vi "Diff Configuration.vi"(8 "error in":errorcluster, 10 "configuration new":T4[](array[typedef]), 11 "configuration old":T4[](array[typedef])) -> (0 "error out":errorcluster, 3 "configuration diff":T1[](array[typedef]))   [LabVIEW 2020, in "Ballard MIL-STD-1553 System Explorer.lvlib" / "Implementation.lvlib" / "Refresh.lvlib"]
uses:
  Refresh.lvlib
  Change Type.ctl
  Symbols.ctl
  MCL Row.ctl
  Scripting/Constants.vi
  Scripting/Ballard MIL-STD-1553 Scripting.lvlib
  Shared/Address.ctl
  Shared/Message Type.ctl
  Shared/Terminal Endpoint.ctl
  Shared/Parameter Definition.ctl
  Shared/Message Definition.ctl
  Shared/1553 Channel.ctl
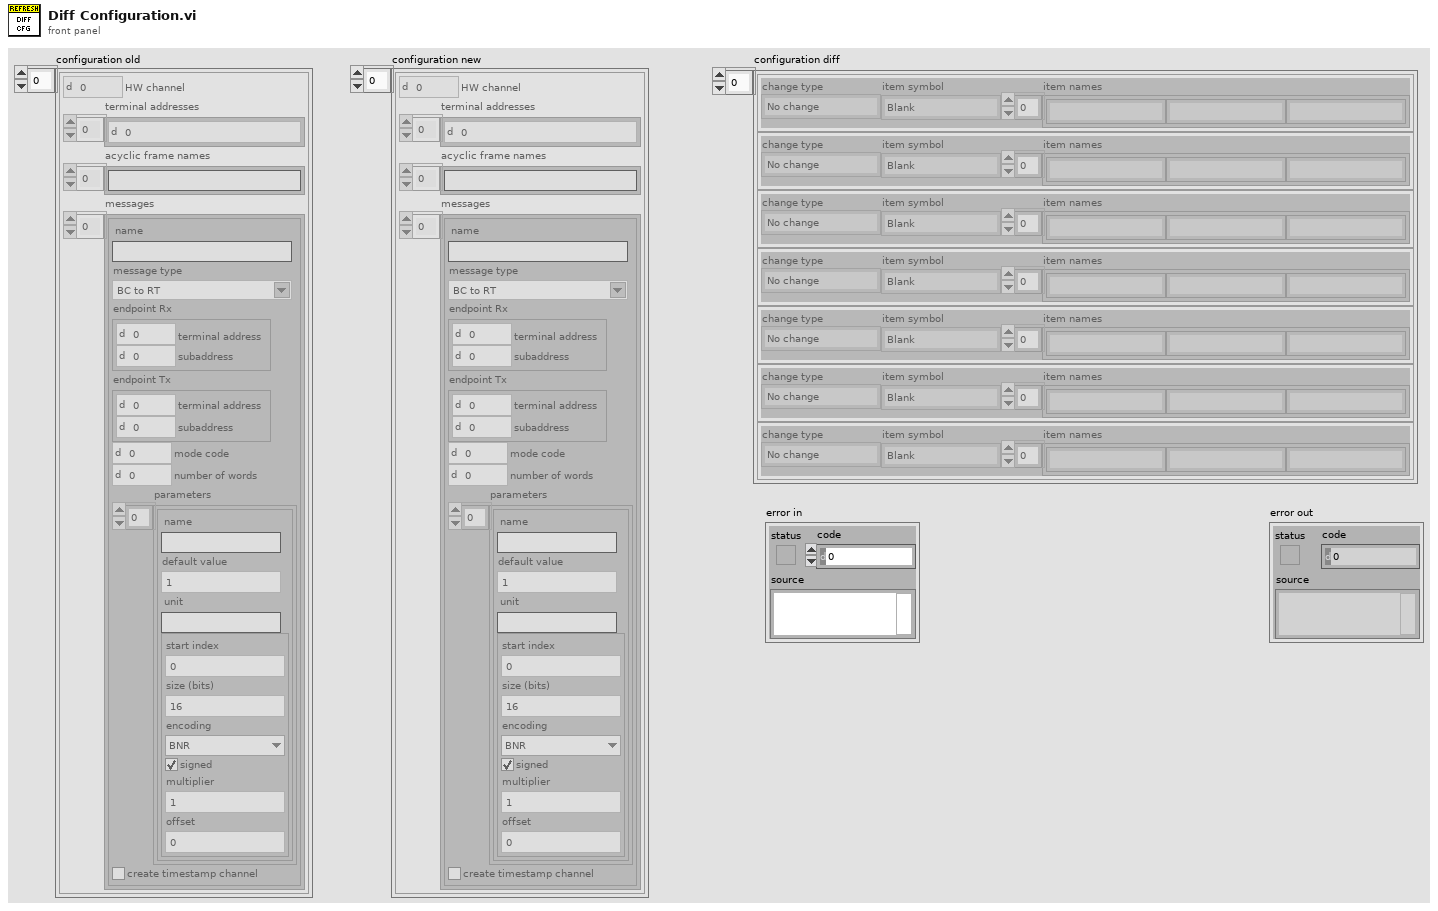
[diagram p1: front panel]
types:
  T1 = typedef "Ballard MIL-STD-1553 System Explorer.lvlib/Implementation.lvlib/Refresh.lvlib/MCL Row.ctl" = cluster{"change type":T2, "item symbol":T3, "item names":string[]}
  T2 = typedef "Ballard MIL-STD-1553 System Explorer.lvlib/Implementation.lvlib/Refresh.lvlib/Change Type.ctl" = enum16{"No change", "Modify", "Add", "Remove"}
  T3 = typedef "Ballard MIL-STD-1553 System Explorer.lvlib/Implementation.lvlib/Refresh.lvlib/Symbols.ctl" = enum16{"Blank", "MIL-STD-1553", "Port", "Remote Terminal", "Subaddress", "Bus Controller", "Acyclic Frame", "Mode Code", "Message", "Parameter", "Item"}
  T4 = typedef "1553 Channel.ctl" = cluster{"HW channel":u16, "terminal addresses":T5[], "acyclic frame names":string[], "messages":T6[]}
  T5 = typedef "Address.ctl" = u16
  T6 = typedef "Message Definition.ctl" = cluster{"name":string, "message type":T7, "endpoint Rx":T8, "endpoint Tx":T8, "mode code":u16, "number of words":u16, "parameters":cluster{"name":string, "default value":dbl, "unit":string, "parameter definition":T9}[], "create timestamp channel":bool}
  T7 = typedef "Message Type.ctl" = string
  T8 = typedef "Terminal Endpoint.ctl" = cluster{"terminal address":T5, "subaddress":T5}
  T9 = typedef "Parameter Definition.ctl" = cluster{"start index":i32, "size (bits)":i32, "encoding":enum16{"BNR", "BCD", "Discrete"}, "signed":bool, "multiplier":dbl, "offset":dbl}
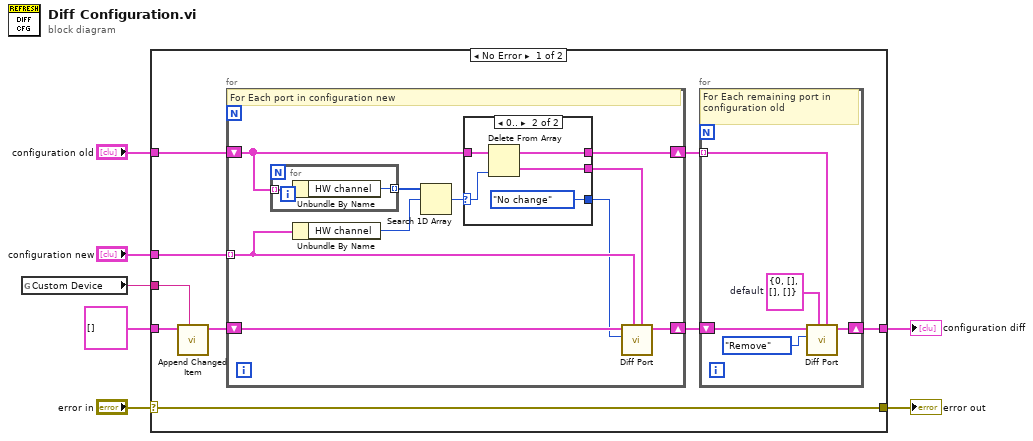
[diagram p0: block diagram]
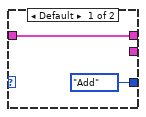
[diagram p2: hidden frame]
diagram:
  n1 = global read "Constants.vi" "Custom Device"() -> (w6:string)
  n2 = case shown="No Error" "error in" {
    selector: "error in" -> [w14 w41]
    tunnel: T1[] [] -> [w16 w42]
    tunnel: w6 -> [w15 _]
    tunnel: [w8 w42] -> w5
    tunnel: [w14 w41] -> w3
    tunnel: "configuration old" -> [w13 _]
    tunnel: "configuration new" -> [w12 _]
    frame No Error {
      n3 = call "Append Changed Item.vi"("item name"=w15, "refresh items in"=w16) -> ("refresh items out"=w11:T1[])  [unwired: 8 in, 1 out]
      n4 = for {
        tunnel: w12 -> [w24] mode=indexing
        shift-right: [w28] -> w9
        shift-left: w13 -> [w29]
        shift-right: [w26] -> w10
        shift-left: w11 -> [w23]
        # "For Each port in configuration new"
        n5 = for {
          tunnel: w29 -> [w40] mode=indexing
          tunnel: [w39] -> w31 mode=indexing
          n6 = Unbundle By Name(w40) -> ("HW channel"=w39:u16)
        }
        n7 = Unbundle By Name(w24) -> ("HW channel"=w30:u16)
        n8 = Search 1D Array(1D array=w31, element=w30) -> (index of element=w27:i32)  [unwired: 1 in]
        n9 = case shown="0.." w27 {
          selector: w27 -> [_ w36]
          tunnel: w29 -> [w33 w38]
          tunnel: [w33 w37] -> w28
          tunnel: [_ w35] -> w25
          tunnel: [Change_Type."Add" ("change type") Change_Type."No change" ("change type")] -> w22
          frame Default {
          }
          frame 0.. {
            n10 = Delete From Array(array=w38, index=w36) -> (deleted portion=w35:T4, array with subset deleted=w37:T4[])  [unwired: 1 in]
          }
        }
        n11 = call "Diff Port.vi"("port old"=w25, "port new"=w24, "change type"=w22, "refresh items in"=w23) -> ("refresh items out"=w26:T1[])  [unwired: 7 in]
      }
      n12 = for {
        shift-right: [w19] -> w8
        shift-left: w10 -> [w21]
        tunnel: w9 -> [w18] mode=indexing
        w17 = T4 {"HW channel"=0, "terminal addresses"=[], "acyclic frame names"=[], "messages"=[]}  # default
        # "For Each remaining port in configuration old"
        n13 = call "Diff Port.vi"("port old"=w18, "port new"=w17, "change type"=Change_Type."Remove", "refresh items in"=w21) -> ("refresh items out"=w19:T1[])  [unwired: 7 in]
      }
    }
    frame Error {
    }
  }
  "configuration diff" <- w5
  "error out" <- w3
